vi "NMD.vi"(8 "error in":errorcluster, 11 "RoI":dbl[][](array[numeric])) -> (0 "error out":errorcluster, 3 "NMD":dbl)   [LabVIEW 2020]
panel:
  out "Waveform Graph":dbl[][](graph)
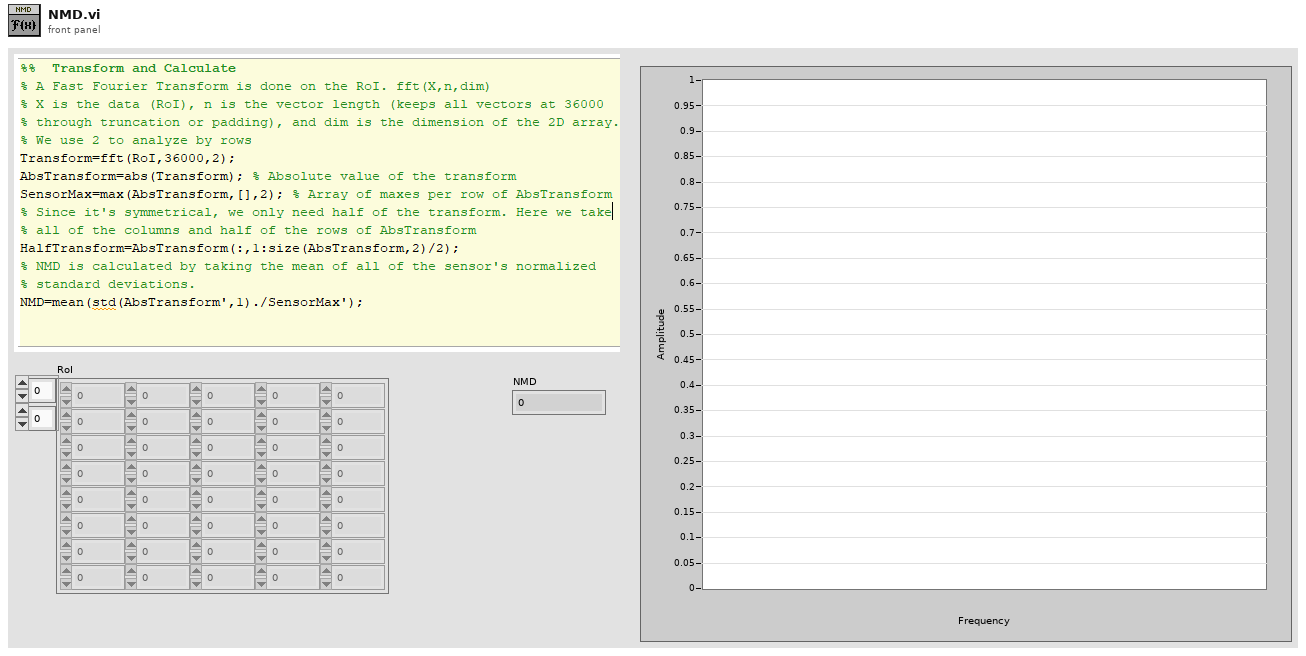
[diagram p1: front panel]
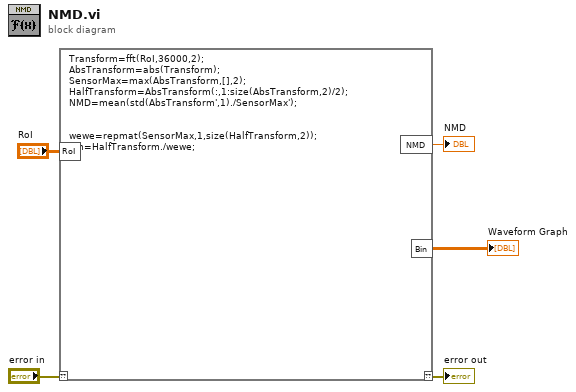
[diagram p0: block diagram]
diagram:
  n1 = script code="Transform=fft(RoI,36000,2); \nAbsTransform=abs(Transform); \nSensorMax=max(AbsTransform,[],2); \nHalfTransform=AbsTransform(:,1:size(AbsTransform,2)/2);\nNMD=mean(std(AbsTransform',1)./SensorMax');\n\n\nwewe=repmat(SensorMax,1,size(HalfTransform,2));\nBin=HalfTransform./wewe;"("??"="error in", "RoI"="RoI") -> ("??"=→"error out":errorcluster, "NMD"=→"NMD":dbl, "Bin"=→"Waveform Graph":dbl[][])
